vi "E17_Tanque.vi"() -> ()   [LabVIEW 2026]
panel:
  out "Y":dbl
  in  "k":dbl
  in  "stop":bool
  out "Tank":dbl(slide) scale=0.0..10.0
  in  "Slide":dbl(slide) scale=0.0..10.0
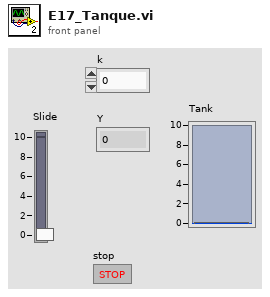
[diagram p1: front panel]
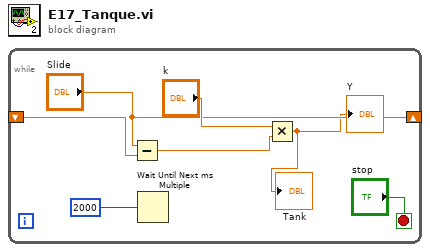
[diagram p0: block diagram]
diagram:
  n1 = while {
    shift-right: ["Slide"] -> _
    shift-left: _ -> [w3]
    stop <- "stop" stop-if-true
    n2 = Subtract(x="Slide", y=w3) -> (x-y=w5:dbl)
    n3 = Wait Until Next ms Multiple(millisecond multiple=u32 2000) -> ()  [unwired: 1 out]
    n4 = Multiply(x="k", y=w5) -> (x*y=→"Y" →"Tank":dbl)
  }
